vi "Create.vi"(8 "error in (no error)":errorcluster) -> (0 "error out":errorcluster, 3 "Bag":refnum<class "Bag.lvclass">)   [LabVIEW 2020, in "Bag.lvclass"]
uses:
  Bag.lvclass
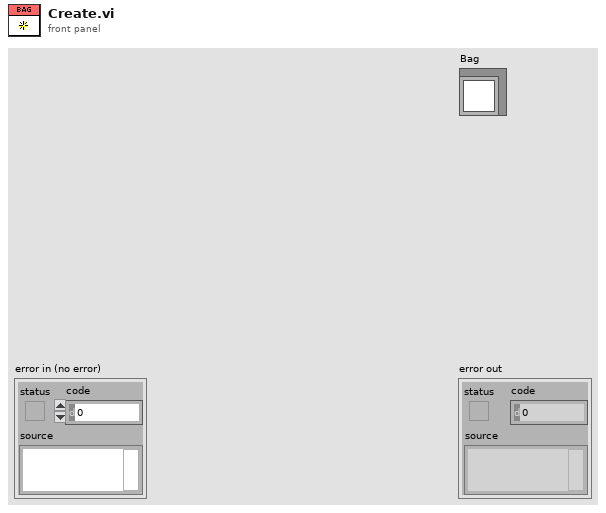
[diagram p1: front panel]
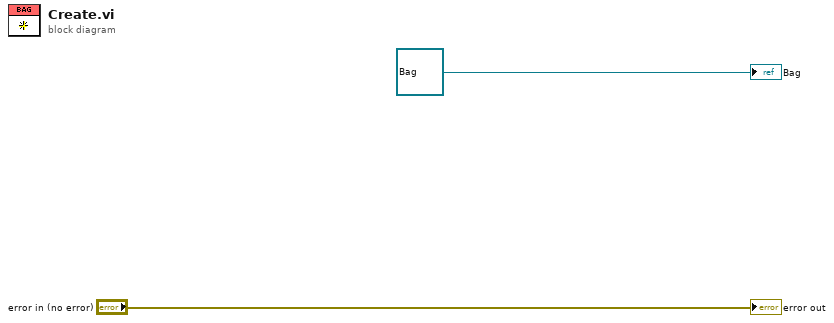
[diagram p0: block diagram]
diagram:
  "error out" <- "error in (no error)"
  "Bag" <- refnum<class "Bag.lvclass"> refnum ("Bag")
